vi "Horizontal Panel Example.vi"() -> ()   [LabVIEW 2013, in "PanelExample.lvclass"]
uses:
  PanelExample.lvclass
  PanelObject/PanelObject.lvclass
  PanelDataNode/Split Mode.ctl
  PanelDataNode/PanelDataNode.lvclass
  PanelLinkNode/PanelLinkNode.lvclass
panel:
  in  "Node*":refnum<data-value>
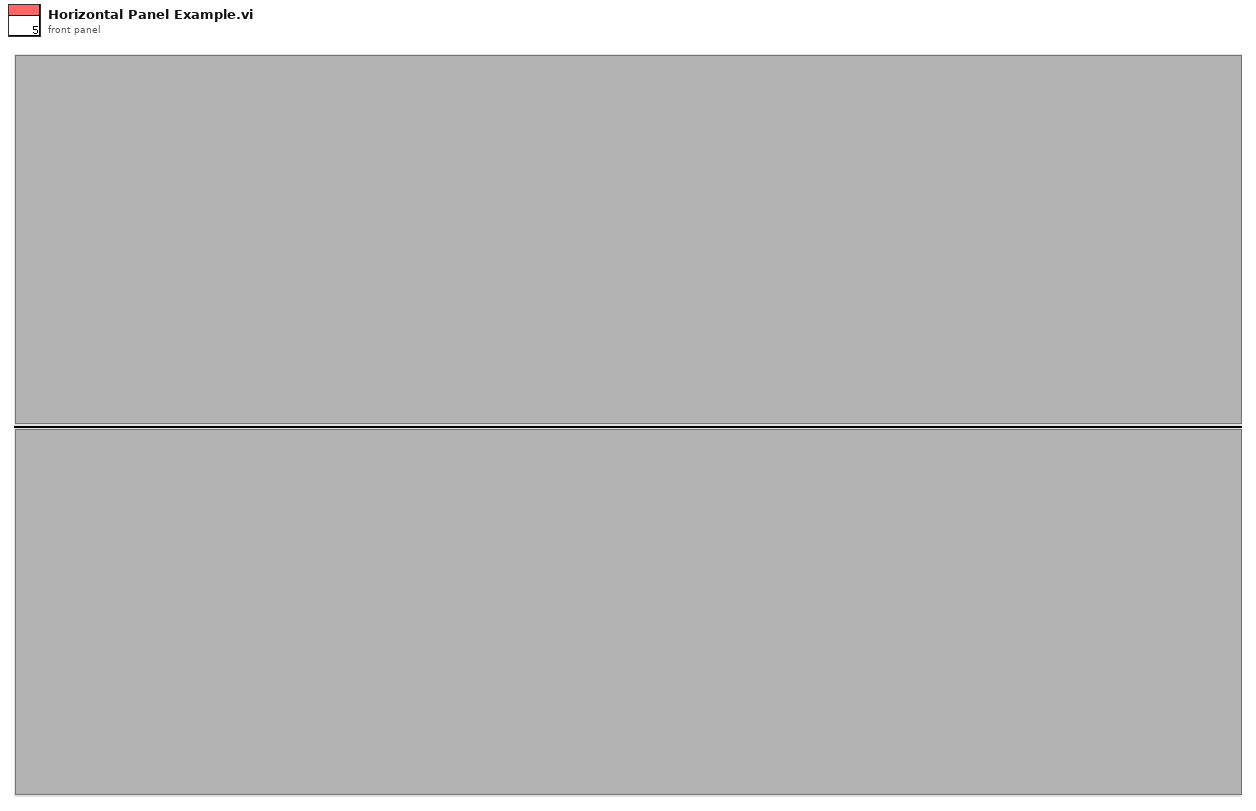
[diagram p1: front panel]
types:
  T1 = typedef "PanelDataNode.lvclass/Split Mode.ctl" = enum16{"Horizontal(up)", "Vertical(left)", "Horizontal(down)", "Vertical(right)"}
  T2 = cluster{"ChildNode*":refnum<data-value>, "Split Mode":T1}
  T3 = cluster{"ChildNode*":refnum<data-value>, "VI*":refnum<vi>}
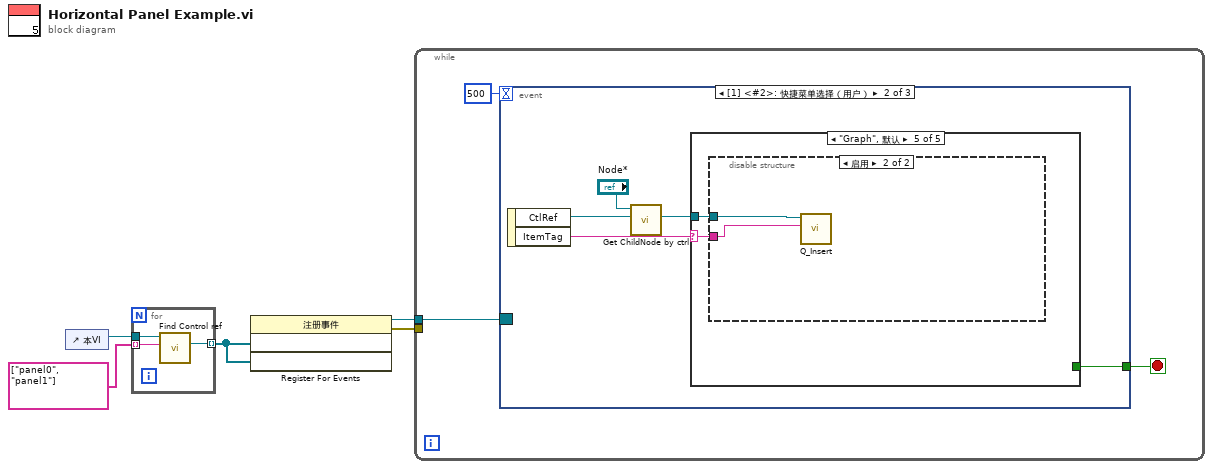
[diagram p0: block diagram]
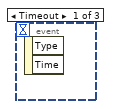
[diagram p2: hidden frame]
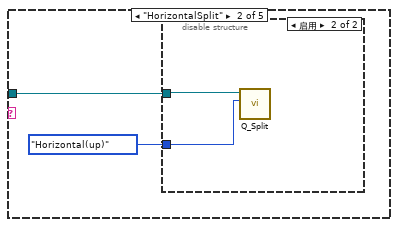
[diagram p4: hidden frame]
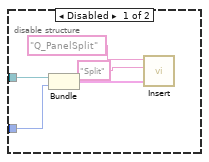
[diagram p5: hidden frame]
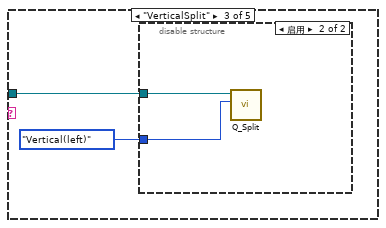
[diagram p6: hidden frame]
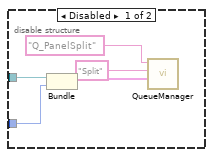
[diagram p7: hidden frame]
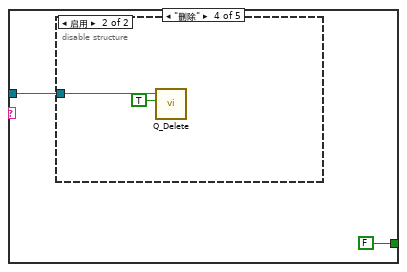
[diagram p8: hidden frame]
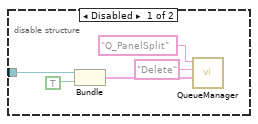
[diagram p9: hidden frame]
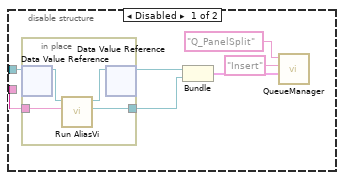
[diagram p10: hidden frame]
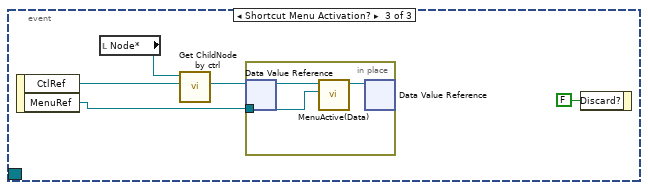
[diagram p11: hidden frame]
diagram:
  n1 = control-ref of="本VI"() -> (w2:refnum<vi>)
  n2 = for {
    tunnel: w2 -> [w8]
    tunnel: string[] ["panel0", "panel1"] -> [w7] mode=indexing
    tunnel: [w6] -> w4 mode=indexing
    n3 = call "Find Control ref.vi"("control name"=w7, "panelvi*"=w8) -> ("ctrl*"=w6:refnum<vi>)  [unwired: 7 in, 2 out]
  }
  n4 = register-events(w4, w4) -> (reference out=w5:refnum<event-registration>, error out=w3:errorcluster)  [unwired: 2 in]
  n5 = while {
    tunnel: w5 -> [w10]
    tunnel: w3 -> [_]
    stop <- w9 stop-if-true
    n6 = event shown="[1] <#2>: 快捷菜单选择（用户）" {
      selector: w10 -> [_ _ _]
      dyn-events: _ -> [_ _ _]
      timeout: 500 -> [_ _ _]
      tunnel: [_ w12 _] -> w9
      event Timeout {
        n7 = event-data() -> ()  [unwired: 1 in, 2 out]
      }
      event Shortcut Menu Selection (User) {
        n8 = event-data() -> ("CtlRef"=w16:refnum<vi>, "ItemTag"=w13:string)  [unwired: 1 in]
        n9 = call "Get ChildNode by ctrl.vi"("ctr*"=w16, "Node*"="Node*") -> ("ChildNode*"=w14:refnum<data-value>)  [unwired: 8 in, 1 out]
        n10 = case shown="\"Graph\", 默认" w13 {
          selector: w13 -> [_ _ _ _ w45]
          tunnel: w14 -> [_ w18 w26 w35 w44]
          tunnel: [_ _ _ FALSE _] -> w12
          frame "假" {
          }
          frame "HorizontalSplit" {
            n11 = disable-structure shown="启用" {
              disable-tunnel: w18 -> [w23 w25]
              disable-tunnel: Split_Mode."Horizontal(up)" ("Split Mode") -> [w22 w24]
              frame Disabled {
                n12 = Bundle("ChildNode*"=w23, "Split Mode"=w22) -> (w21:T2)  [unwired: 1 in]
                n13 = call "Insert.vi"("Data"=w21, "Event"="Split", "QueueName"="Q_PanelSplit") -> ()  [unwired: 7 in, 2 out]
              }
              frame Enabled {
                n14 = call "Q_Split.vi"("Split Mode"=w24, "ChildNode*"=w25) -> ()  [unwired: 9 in, 1 out]
              }
            }
          }
          frame "VerticalSplit" {
            n15 = disable-structure shown="启用" {
              disable-tunnel: Split_Mode."Vertical(left)" ("Split Mode") -> [w32 w34]
              disable-tunnel: w26 -> [w31 w33]
              frame Disabled {
                n16 = Bundle("ChildNode*"=w31, "Split Mode"=w32) -> (w28:T2)  [unwired: 1 in]
                n17 = call-poly "QueueManager.vi"("Data"=w28, "Event"="Split", "QueueName"="Q_PanelSplit") -> ()  [unwired: 7 in, 2 out]
              }
              frame Enabled {
                n18 = call "Q_Split.vi"("Split Mode"=w34, "ChildNode*"=w33) -> ()  [unwired: 9 in, 1 out]
              }
            }
          }
          frame "删除" {
            n19 = disable-structure shown="启用" {
              disable-tunnel: w35 -> [w41 w43]
              frame Disabled {
                n20 = Bundle("ChildNode*"=w41, TRUE) -> (w40:cluster{"ChildNode*":refnum<data-value>, bool})  [unwired: 1 in]
                n21 = call-poly "QueueManager.vi"("Data"=w40, "Event"="Delete", "QueueName"="Q_PanelSplit") -> ()  [unwired: 7 in, 2 out]
              }
              frame Enabled {
                n22 = call "Q_Delete.vi"("CloseVI?(T)"=TRUE, "ChildNode*"=w43) -> ()  [unwired: 9 in, 1 out]
              }
            }
          }
          frame "Graph", Default {
            n23 = disable-structure shown="启用" {
              disable-tunnel: w45 -> [w49 w57]
              disable-tunnel: w44 -> [w48 w58]
              frame Disabled {
                n24 = in-place {
                  in-place-border: w49 -> [w56]
                  in-place-border: [w53] -> w46
                  n25 = in-place-dvr #1(w48) -> (w55:refnum<class "PanelDataNode.lvclass">)  [unwired: 1 out]
                  n26 = call-dynamic "Run AliasVi.vi"("Vi Alias"=w56, "PanelDataNode 输入"=w55) -> ("VI*"=w53:refnum<vi>, "PanelDataNode 输出"=w54:refnum<class "PanelDataNode.lvclass">)  [unwired: 7 in, 1 out]
                  n27 = in-place-dvr #1(w54) -> (w47:refnum<data-value>)  [unwired: 1 out]
                }
                n28 = Bundle("ChildNode*"=w47, "VI*"=w46) -> (w52:T3)  [unwired: 1 in]
                n29 = call-poly "QueueManager.vi"("Data"=w52, "Event"="Insert", "QueueName"="Q_PanelSplit") -> ()  [unwired: 7 in, 2 out]
              }
              frame Enabled {
                n30 = call "Q_Insert.vi"("Vi Alias"=w57, "ChildNode*"=w58) -> ()  [unwired: 9 in, 1 out]
              }
            }
          }
        }
      }
      event Shortcut Menu Activation? {
        n31 = event-data() -> ("CtlRef"=w63:refnum<vi>, "MenuRef"=w60:refnum<k9>)  [unwired: 1 in]
        n32 = local read "Node*"() -> (w62:refnum<data-value>)
        n33 = call "Get ChildNode by ctrl.vi"("ctr*"=w63, "Node*"=w62) -> ("ChildNode*"=w61:refnum<data-value>)  [unwired: 8 in, 1 out]
        n34 = in-place {
          in-place-border: w60 -> [w65]
          n35 = in-place-dvr #2(w61) -> (w66:refnum<class "PanelDataNode.lvclass">)  [unwired: 1 out]
          n36 = call-dynamic "MenuActive(Data).vi"("菜单引用"=w65, "PanelDataNode 输入"=w66) -> ("PanelDataNode 输出"=w64:refnum<class "PanelDataNode.lvclass">)  [unwired: 7 in, 2 out]
          n37 = in-place-dvr #2(w64) -> ()  [unwired: 2 out]
        }
        n38 = event-data("Discard?"=FALSE ("放弃？")) -> ()  [unwired: 1 in, 1 out]
      }
    }
  }
